vi "ArcadeDrivePoly.vi"   [LabVIEW 2013]
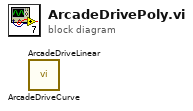
[diagram p0: block diagram]
diagram:
  n1 = call "ArcadeDriveCurve.vi"() -> ()  [unwired: 10 in, 2 out]
  n2 = call "ArcadeDriveLinear.vi"() -> ()  [unwired: 10 in, 2 out]
